vi "test_ScopeInstruments_InitializeSessionsWithUnregisteredSessionsReserved_RemoteSessionsInitialized.vi"(8 "error in":errorcluster) -> (0 "error out":errorcluster, 2 "result":string, 3 "pass":bool)   [LabVIEW 2020, in "MeasurementServerTests.lvlib"]
uses:
  MeasurementServerTests.lvlib
  Runtime/Sessions/niScope Sessions/niScope Sessions.lvlib
  c4a911aa-80ea-4246-aa9a-6d8f5dfeb207.vi
  Runtime/Sessions/niScope Sessions/Initialize Sessions - NSess.vi
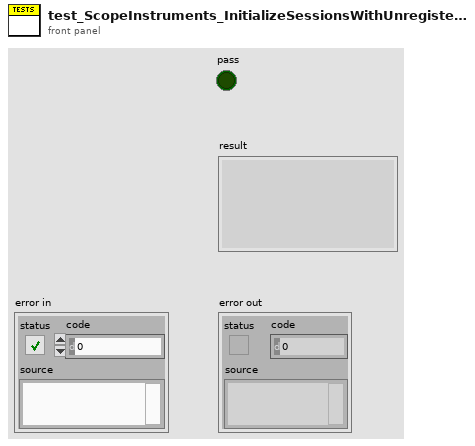
[diagram p1: front panel]
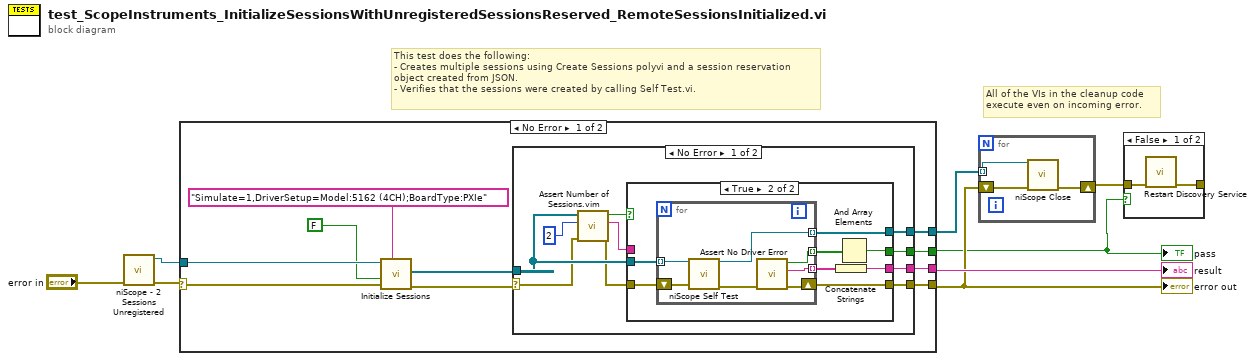
[diagram p0: block diagram]
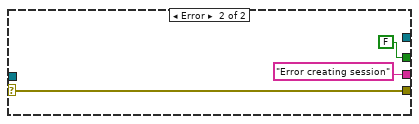
[diagram p3: hidden frame]
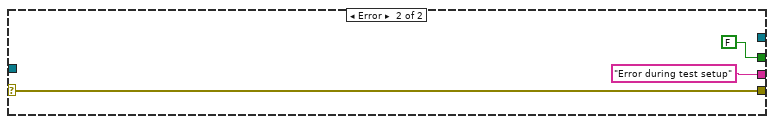
[diagram p4: hidden frame]
diagram:
  # "All of the VIs in the cleanup code\nexecute even on incoming error."
  # "This test does the following:\n- Creates multiple sessions using Create Sessions polyvi and a session reservation\nobject created from JSON.\n- Verifies that the sessions were created by calling Self Test.vi."
  n1 = call "niScope - 2 Sessions Unregistered.vi"("error in"="error in") -> ("error out"=w4:errorcluster, "session reservation out"=w3:refnum<class "Session Reservation.lvclass">)  [unwired: 9 in]
  n2 = case shown="No Error" w4 {
    selector: w4 -> [w12 w51]
    tunnel: [w17 w51] -> w6
    tunnel: [w18 FALSE] -> w1
    tunnel: [w16 "Error during test setup" ("f")] -> w8
    tunnel: [w15 _] -> w7
    tunnel: w3 -> [w11 _]
    frame No Error {
      n3 = call-poly "Initialize Sessions.vi"("option string"="Simulate=1,DriverSetup=Model:5162 (4CH);BoardType:PXIe", "error in"=w12, "reset"=FALSE, "session reservation in"=w11) -> ("error out"=w10:errorcluster, "sessions"=w13:refnum<k15>[])  [unwired: 4 in, 2 out]
      n4 = case shown="No Error" w10 {
        selector: w10 -> [w22 w49]
        tunnel: [w28 FALSE] -> w18
        tunnel: [w26 w49] -> w17
        tunnel: [w27 "Error creating session"] -> w16
        tunnel: w13 -> [w24 _]
        tunnel: [w25 _] -> w15
        frame No Error {
          n5 = call "Assert Number of Sessions.vim"("error in"=w22, "expected number of sessions"=2, "sessions"=w24) -> ("error out"=w23:errorcluster, "result"=w19:string, "pass"=w20:bool)  [unwired: 6 in]
          n6 = case shown="True" w20 {
            selector: w20 -> [w29 _]
            tunnel: [w29 w35] -> w28
            tunnel: [w30 w33] -> w27
            tunnel: [w31 w40] -> w26
            tunnel: [w32 w39] -> w25
            tunnel: w24 -> [w32 w38]
            tunnel: w23 -> [w31 w37]
            tunnel: w19 -> [w30 _]
            frame False {
            }
            frame True {
              n7 = for {
                tunnel: [w47] -> w36 mode=indexing
                tunnel: [w46] -> w34 mode=indexing
                tunnel: [w44] -> w39 mode=indexing
                tunnel: w38 -> [w42] mode=indexing
                shift-right: [w45] -> w40
                shift-left: w37 -> [w41]
                n8 = call <instrlib>:"niScope Self Test.vi"("instrument handle"=w42, "error in"=w41) -> ("instrument handle out"=w44:refnum<k15>, "error out"=w43:errorcluster)  [unwired: 10 in, 2 out]
                n9 = call "Assert No Driver Error.vi"("error in"=w43) -> ("error out"=w45:errorcluster, "result"=w46:string, "pass?"=w47:bool)  [unwired: 8 in]
              }
              n10 = Concatenate Strings(w34) -> (w33:string)
              n11 = And Array Elements(Boolean array=w36) -> (logical AND=w35:bool)
            }
          }
        }
        frame Error {
        }
      }
    }
    frame Error {
    }
  }
  "error out" <- w6
  "pass" <- w1
  "result" <- w8
  n12 = for {
    tunnel: w7 -> [w56] mode=indexing
    shift-right: [w55] -> w2
    shift-left: w6 -> [w54]
    n13 = call <instrlib>:"niScope Close.vi"("instrument handle"=w56, "error in"=w54) -> ("error out"=w55:errorcluster)  [unwired: 13 in]
  }
  n14 = case shown="False" w1 {
    tunnel: w2 -> [w58 _]
    tunnel: [w57 _] -> _
    frame False {
      n15 = call "Restart Discovery Service.vi"("error in"=w58) -> ("error out"=w57:errorcluster)  [unwired: 10 in]
    }
    frame True {
    }
  }
